vi "Init Bfr Rx - Create Buffer.vi"(8 "error in (no error)":errorcluster, 11 "Rx Loop Data in":T1 {"Data Buffer" format="%016x"}) -> (0 "error out":errorcluster, 3 "Rx Loop Data out":T1 {"Data Buffer" format="%016x"})   [LabVIEW 2016, in "UDP-Custom-Device Engine.lvlib"]
uses:
  UDP-Custom-Device Engine.lvlib
  Types/Engine - Buffered Rx Loop Data.ctl
  Shared/Types/Shared - Header Details.ctl
  Shared/Types/Shared - Buffered.PacketInfo.ctl
  <vilib>/NI/NIVS Inline Async API/_Data Access Engine/Data Access Engine/Types/Read.DVR.ctl
  <vilib>/NI/NIVS Inline Async API/_Data Access Engine/Access Type Classes/Read/Read.lvclass
  <vilib>/NI/NIVS Inline Async API/_Data Access Engine/Data Access Engine/Types/Write.DVR.ctl
  <vilib>/NI/NIVS Inline Async API/_Data Access Engine/Access Type Classes/Write/Write.lvclass
  <vilib>/NI/NIVS Inline Async API/_Data Access Engine/Access Type Classes/Write/Write.lvclass/Write.ctl
  <vilib>/NI Veristand/VeriStand Data/Library/Pointer Operations/Pointer.Write (String).vi
  <vilib>/NI/NIVS Inline Async API/_Data Access Engine/Data Access Engine/Methods/Write.Data.vi
  <vilib>/NI/NIVS Inline Async API/_Data Access Engine/Access Type Classes/Write/Write.ProcessData.vi
  <vilib>/NI Veristand/VeriStand Data/Library/VeriStand Data.lvlib
  <vilib>/NI/NIVS Inline Async API/_Data Access Engine/Data Access Engine/Data Access Engine.lvclass
  Shared/UDP-Custom-Device Shared.lvlib
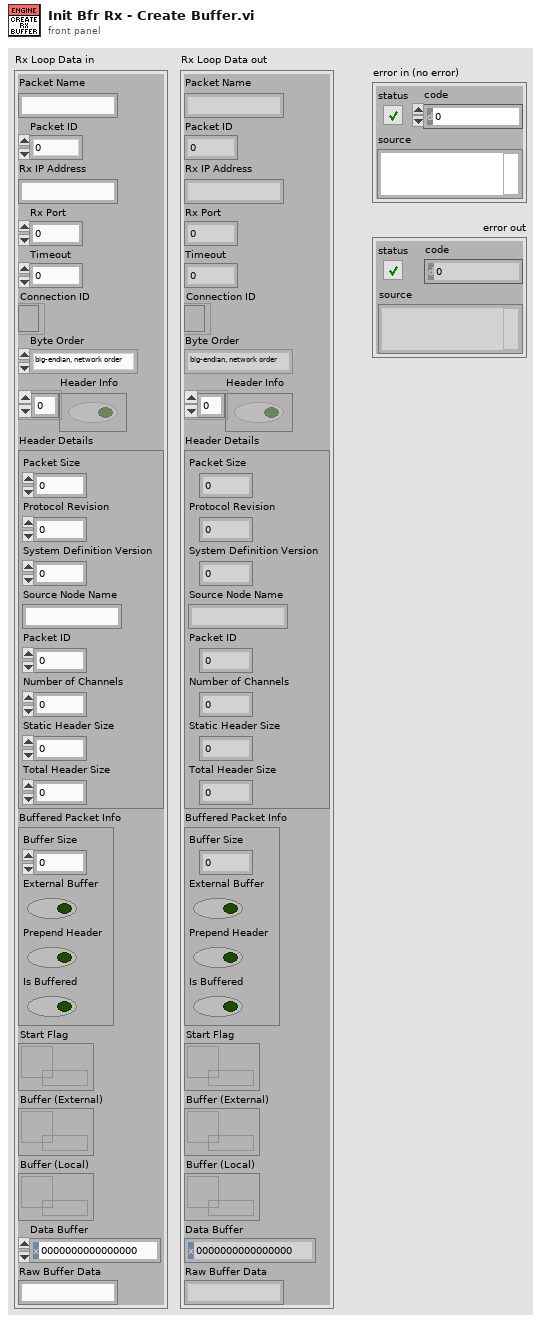
[diagram p1: front panel]
types:
  T1 = typedef "UDP-Custom-Device Engine.lvlib/Engine - Buffered Rx Loop Data.ctl" = cluster{"Packet Name":string, "Packet ID":i32, "Rx IP Address":string, "Rx Port":i32, "Timeout":i32, "Connection ID":refnum<k16>, "Byte Order":enum16{"big-endian, network order", "native, host order", "little-endian"}, "Header Info":bool[], "Header Details":T2, "Buffered Packet Info":T3, "Start Flag":T4, "Buffer (External)":T4, "Buffer (Local)":T5, "Data Buffer":u64, "Raw Buffer Data":string}
  T2 = typedef "UDP-Custom-Device Shared.lvlib/Shared - Header Details.ctl" = cluster{"Packet Size":u16, "Protocol Revision":u8, "System Definition Version":u64, "Source Node Name":string, "Packet ID":u32, "Number of Channels":u32, "Static Header Size":u16, "Total Header Size":u16}
  T3 = typedef "UDP-Custom-Device Shared.lvlib/Shared - Buffered.PacketInfo.ctl" = cluster{"Buffer Size":i32, "External Buffer":bool, "Prepend Header":bool, "Is Buffered":bool}
  T4 = typedef "Data Access Engine.lvlib/Data Access Engine.lvclass/Read.DVR.ctl" = refnum<data-value>
  T5 = typedef "Data Access Engine.lvlib/Data Access Engine.lvclass/Write.DVR.ctl" = refnum<data-value>
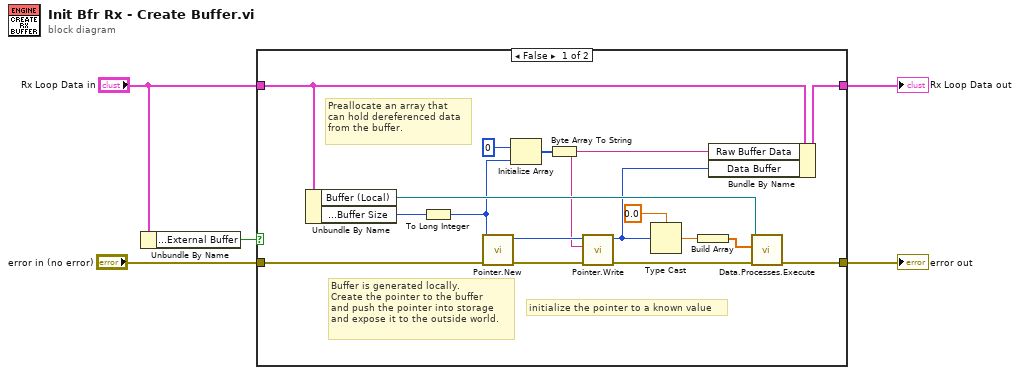
[diagram p0: block diagram]
diagram:
  n1 = Unbundle By Name("Rx Loop Data in") -> ("Buffered Packet Info.External Buffer"=w1:bool)
  n2 = case shown="False" w1 {
    tunnel: "error in (no error)" -> [w21 w23]
    tunnel: [w11 w23] -> w4
    tunnel: "Rx Loop Data in" -> [w20 w24]
    tunnel: [w19 w24] -> w3
    frame False {
      # "initialize the pointer to a known value"
      # "Preallocate an array that\ncan hold dereferenced data\nfrom the buffer."
      # "Buffer is generated locally.\nCreate the pointer to the buffer\nand push the pointer into storage\nand expose it to the outside world."
      n3 = Unbundle By Name(w20) -> ("Buffer (Local)"=w17:T5, "Buffered Packet Info.Buffer Size"=w22:i32)
      n4 = To Long Integer(number=w22) -> (32bit integer=w16:i32)
      n5 = call <vilib>:"Pointer.New.vi"("error in (no error)"=w21, "size in bytes"=w16) -> ("error out"=w7:errorcluster, "pointer"=w10:u64)  [unwired: 8 in]
      n6 = Initialize Array(u8 0, w16) -> (w14:u8[])
      n7 = Byte Array To String(unsigned byte array=w14) -> (string=w9:string)
      n8 = call-poly <vilib>:"Pointer.Write.vi"("error in (no error)"=w7, "string in"=w9, "pointer in"=w10) -> ("error out"=w6:errorcluster, "pointer out"=w8:u64)  [unwired: 6 in, 1 out]
      n9 = Type Cast(type=0.0, x=w8) -> (*(type *) &x=w13:dbl)
      n10 = Build Array(w13) -> (w12:dbl[])
      n11 = Bundle By Name(cluster=w20, "Raw Buffer Data"=w9, "Data Buffer"=w8) -> (w19:T1)
      n12 = call-poly <vilib>:"Data.Processes.Execute.vi"("error in (no error)"=w6, "Values"=w12, "Ref"=w17) -> ("error out"=w11:errorcluster)  [unwired: 8 in]
    }
    frame True {
    }
  }
  "Rx Loop Data out" <- w3
  "error out" <- w4
